vi "Translator.GatherControls.Prepare.vi"(8 "error in":errorcluster, 9 "root":string, 10 "Controls in":refnum<vi>[](array[refnum])) -> (0 "error out":errorcluster, 2 "Controls out":T1[](array[typedef]))   [LabVIEW 2019, in "Tools.lvlib"]
uses:
  Tools.lvlib
  Translator.ControlData.ctl
  Translator.ControlTypes.ctl
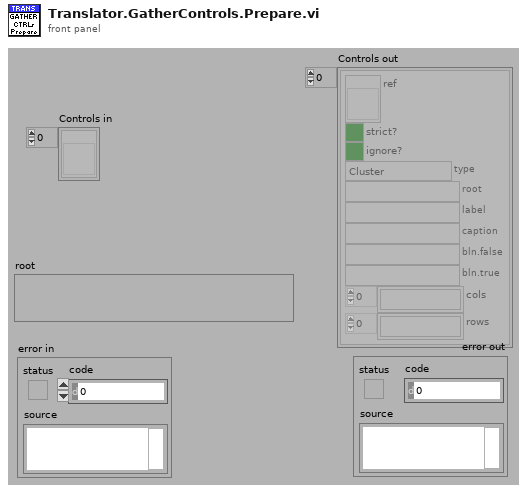
[diagram p1: front panel]
types:
  T1 = typedef "Tools.lvlib/Translator.ControlData.ctl" = cluster{"ref":refnum<vi>, "strict?":bool, "ignore?":bool, "type":T2, "root":string, "label":string, "caption":string, "bln.false":string, "bln.true":string, "cols":string[], "rows":string[]}
  T2 = typedef "Tools.lvlib/Translator.ControlTypes.ctl" = enum16{"Cluster", "Array", "Boolean", "Ring", "String", "Tab", "Listbox", "Multicolumn listbox", "Table", "Other"}
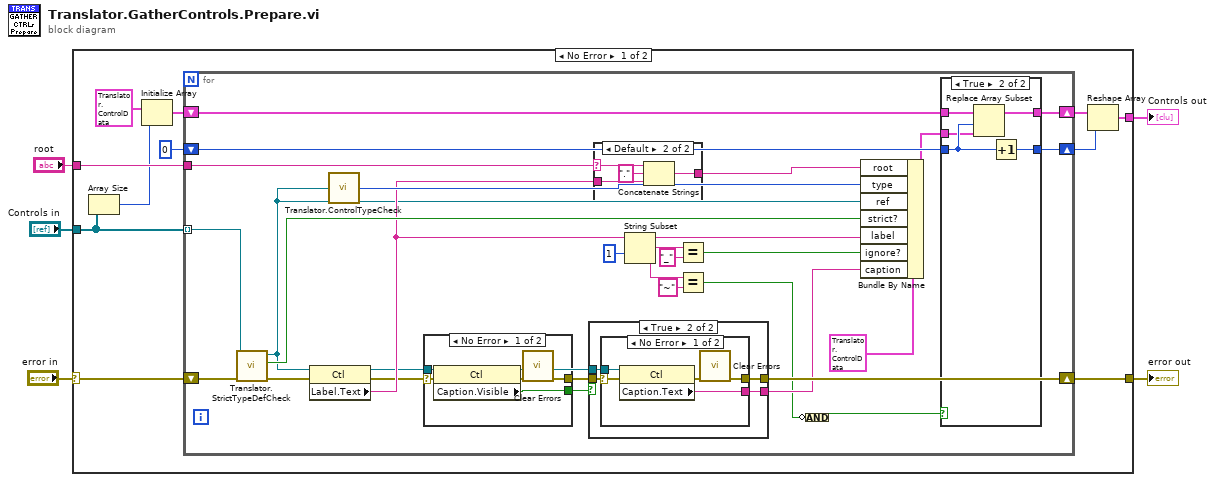
[diagram p0: block diagram]
diagram:
  n1 = case shown="No Error" "error in" {
    selector: "error in" -> [w15 w74]
    tunnel: "Controls in" -> [w13 _]
    tunnel: [w16 w74] -> w4
    tunnel: [w6 _] -> w3
    tunnel: "root" -> [w14 _]
    frame No Error {
      n2 = Array Size(array=w13) -> (size(s)=w11:i32)
      n3 = Initialize Array(T1 {"ref"=refnum, "strict?"=FALSE, "ignore?"=FALSE, "type"=enum."Cluster", "root"="", "label"="", "caption"="", "bln.false"="", "bln.true"="", "cols"=[], "rows"=[]} ("ControlData"), w11) -> (w10:T1[])
      n4 = for {
        shift-right: [w42] -> w16
        shift-left: w15 -> [w41]
        tunnel: w13 -> [w38] mode=indexing
        tunnel: w14 -> [w36]
        shift-right: [w32] -> w8
        shift-left: w10 -> [w34]
        shift-right: [w31] -> w7
        shift-left: 0 -> [w33]
        n5 = call "Translator.StrictTypeDefCheck.vi"("error in (no error)"=w41, "Ctl Refnum in"=w38) -> ("error out"=w39:errorcluster, "Strict Type def?"=w40:bool, "Ctl Refnum out"=w23:refnum<vi>)  [unwired: 7 in]
        n6 = property class="Ctl"(reference=w23, error in=w39) -> (reference out=w24:refnum<vi>, error out=w25:errorcluster, "Label.Text"=w27:string)
        n7 = call "Translator.ControlTypeCheck.vi"("control ref"=w23) -> ("control type"=w43:T2)
        n8 = case shown="No Error" w25 {
          selector: w25 -> [w60 w61]
          tunnel: [w57 w61] -> w18
          tunnel: w24 -> [w58 _]
          tunnel: [w56 _] -> w17
          frame No Error {
            n9 = property class="Ctl"(reference=w58, error in=w60) -> (error out=w59:errorcluster, "Caption.Visible"=w56:bool)  [unwired: 1 out]
            n10 = call <vilib>:"Clear Errors.vi"("error in (no error)"=w59) -> ("error out"=w57:errorcluster)  [unwired: 5 in, 1 out]
          }
          frame Error {
          }
        }
        n11 = case shown="True" w17 {
          tunnel: [w45 w49] -> w42
          tunnel: [_ w48] -> w35
          tunnel: w24 -> [_ w47]
          tunnel: w18 -> [w45 w46]
          frame False {
          }
          frame True {
            n12 = case shown="No Error" w46 {
              selector: w46 -> [w54 w55]
              tunnel: [w50 _] -> w48
              tunnel: [w51 w55] -> w49
              tunnel: w47 -> [w52 _]
              frame No Error {
                n13 = property class="Ctl"(reference=w52, error in=w54) -> (error out=w53:errorcluster, "Caption.Text"=w50:string)  [unwired: 1 out]
                n14 = call <vilib>:"Clear Errors.vi"("error in (no error)"=w53) -> ("error out"=w51:errorcluster)  [unwired: 5 in, 1 out]
              }
              frame Error {
              }
            }
          }
        }
        n15 = case shown="Default" w36 {
          selector: w36 -> [_ w70]
          tunnel: [w69 w73] -> w37
          tunnel: w27 -> [w69 w72]
          frame "" {
          }
          frame Default {
            n16 = Concatenate Strings(w70, "." ("string"), w72) -> (w73:string)
          }
        }
        n17 = String Subset(string=w27, length (rest)=1 ("length (rest)")) -> (substring=w20:string)  [unwired: 1 in]
        n18 = Equal?(x=w20, y="_") -> (x = y?=w26:bool)
        n19 = Equal?(x=w20, y="~") -> (x = y?=w19:bool)
        n20 = Compound Arithmetic op=AND(invert w19) -> (w22:bool)
        n21 = Bundle By Name(cluster=T1 {"ref"=refnum, "strict?"=FALSE, "ignore?"=FALSE, "type"=enum."Cluster", "root"="", "label"="", "caption"="", "bln.false"="", "bln.true"="", "cols"=[], "rows"=[]} ("ControlData"), "root"=w37, "type"=w43, "ref"=w23, "strict?"=w40, "label"=w27, "ignore?"=w26, "caption"=w35) -> (w30:T1)
        n22 = case shown="True" w22 {
          tunnel: w34 -> [w62 w68]
          tunnel: w33 -> [w63 w66]
          tunnel: [w62 w67] -> w32
          tunnel: [w63 w65] -> w31
          tunnel: w30 -> [_ w64]
          frame False {
          }
          frame True {
            n23 = Replace Array Subset(array=w68, new element=w64, index=w66) -> (w67:T1[])
            n24 = Increment(x=w66) -> (x+1=w65:i32)
          }
        }
      }
      n25 = Reshape Array(w8, w7) -> (w6:T1[])
    }
    frame Error {
    }
  }
  "Controls out" <- w3
  "error out" <- w4
